vi "ziModGetIntegerData.vi"(8 "Error In":errorcluster, 10 "ModResults":T3, 11 "ModHandle In":T7 {"ModHandle" format="0x%08x"; "Conn" format="0x%08x"}) -> (0 "Error Out":errorcluster, 1 "ModIntegerDataGrid":T1[](array[typedef]), 2 "ModIntegerData":T2[](array[typedef]), 3 "ModHandle Out":T7 {"ModHandle" format="0x%08x"; "Conn" format="0x%08x"}, 4 "Value":i64[](array[numeric]))   [LabVIEW 2009, in "Zurich Instruments LabOne.lvlib"]
doc: "Use this vi to get IntegerData from a ModResult returned from ziModGetNextNode.vi. It return an array of IntegerData."
uses:
  <instrlib>/Zurich Instruments LabOne/Zurich Instruments LabOne.lvlib
  <instrlib>/Zurich Instruments LabOne/Public/Modules/ziTypeModHandle.ctl
  <instrlib>/Zurich Instruments LabOne/Public/Modules/ziTypeModResults.ctl
  <instrlib>/Zurich Instruments LabOne/Public/Data/ziTypePollType.ctl
  <instrlib>/Zurich Instruments LabOne/Public/Modules/ziTypeModSWTriggerHeader.ctl
  <instrlib>/Zurich Instruments LabOne/Public/Modules/ziTypeModSweeperHeader.ctl
  <instrlib>/Zurich Instruments LabOne/Public/Data/ziTypeIntegerDataTS.ctl
  <instrlib>/Zurich Instruments LabOne/Public/Data/ziTypeIntegerDataTSGrid.ctl
  <instrlib>/Zurich Instruments LabOne/Private/ziLV32.dll
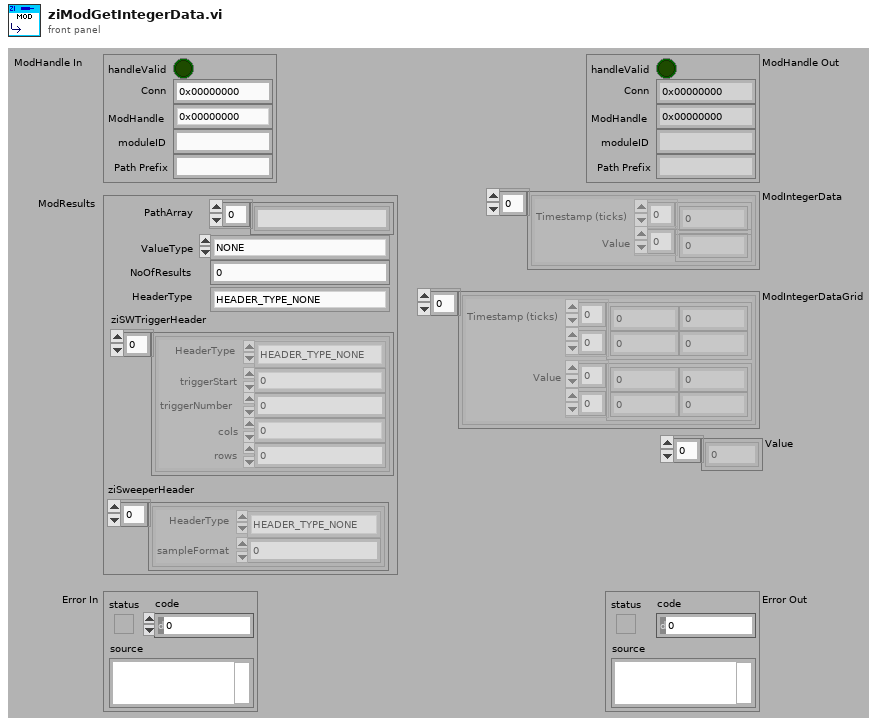
[diagram p1: front panel]
types:
  T1 = typedef "ziTypeIntegerDataTSGrid.ctl" = cluster{"Timestamp (ticks)":u64[][], "Value":i64[][]}
  T2 = typedef "Zurich Instruments LabOne.lvlib/ziTypeIntegerDataTS.ctl" = cluster{"Timestamp (ticks)":u64[], "Value":i64[]}
  T3 = typedef "Zurich Instruments LabOne.lvlib/ziTypeModResults.ctl" = cluster{"PathArray":string[], "ValueType":T4, "NoOfResults":u64, "HeaderType":enum16{"HEADER_TYPE_NONE", "HEADER_TYPE_SWTRIGGER", "HEADER_TYPE_SWEEPER"}, "ziSWTriggerHeader":T5[], "ziSweeperHeader":T6[]}
  T4 = typedef "Zurich Instruments LabOne.lvlib/ziTypePollType.ctl" = enum16{"NONE", "DOUBLE_DATA", "INTEGER_DATA", "DEMOD_SAMPLE", "SCOPE_WAVE_HF2", "AUXIN_SAMPLE", "DIO_SAMPLE", "BYTE_ARRAY", "PWA_WAVE", "9", "10", "11", "12", "13", "14", "15", "TREE_CHANGE_DEPRI", "17", "ERROR", "19", "20", "21", "22", "23", "24", "25", "26", "27", "28", "29", "30", "31", "DOUBLE_DATA_TS", "INTEGER_DATA_TS", "34", "SCOPE_WAVE", "36", "37", "BYTE_ARRAY_TS", "39", "40", "41", "42", "43", "44", "45", "CNT_DATA", "47", "TREE_CHANGE", "49", "50", "51", "52", "53", "54", "55", "56", "57", "58", "59", "60", "61", "62", "63", "SWEEPER_DATA", "SPECTRUM_DATA", "ADVISOR_DATA", "67", "IMP_DATA"}
  T5 = typedef "Zurich Instruments LabOne.lvlib/ziTypeModSWTriggerHeader.ctl" = cluster{"HeaderType":enum8{"HEADER_TYPE_NONE", "HEADER_TYPE_SWTRIGGER", "HEADER_TYPE_SWEEPER"}, "triggerStart":u64, "triggerNumber":u64, "cols":u32, "rows":u32}
  T6 = typedef "Zurich Instruments LabOne.lvlib/ziTypeModSweeperHeader.ctl" = cluster{"HeaderType":enum8{"HEADER_TYPE_NONE", "HEADER_TYPE_SWTRIGGER", "HEADER_TYPE_SWEEPER"}, "sampleFormat":u8}
  T7 = typedef "Zurich Instruments LabOne.lvlib/ziTypeModHandle.ctl" = cluster{"handleValid":bool, "Conn":u64, "ModHandle":u64, "moduleID":string, "Path Prefix":string}
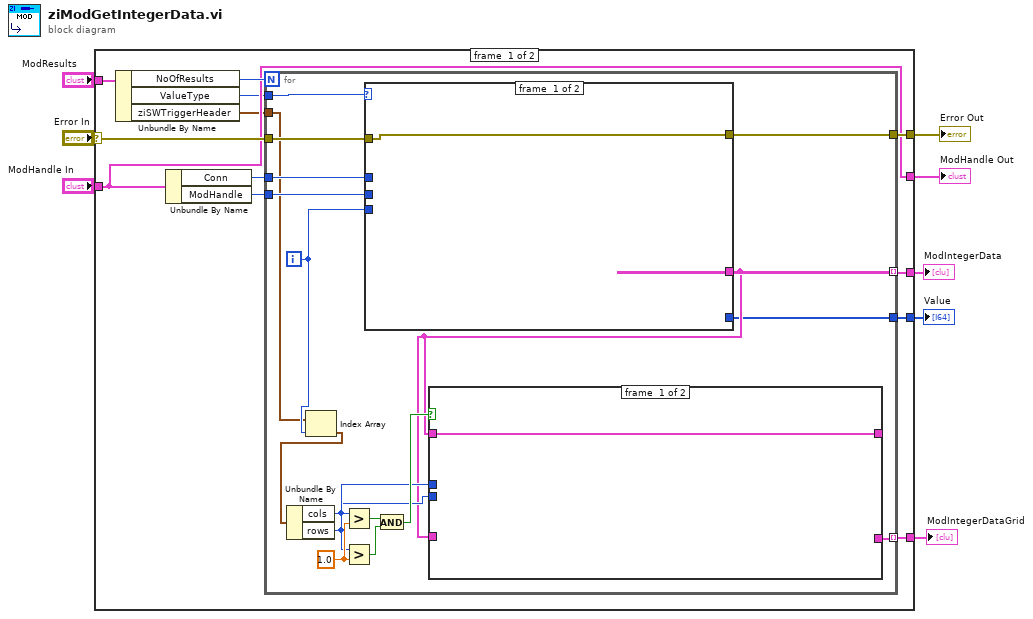
[diagram p0: block diagram]
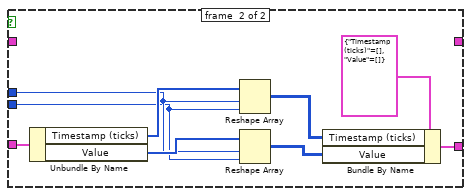
[diagram p2: hidden frame]
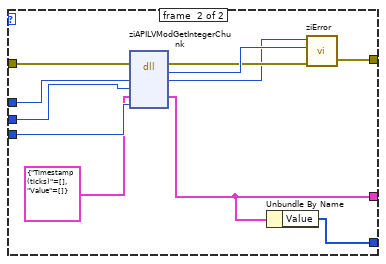
[diagram p3: hidden frame]
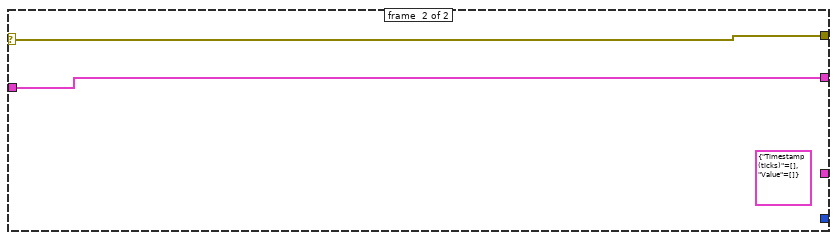
[diagram p4: hidden frame]
diagram:
  n1 = case shown="No Error" "Error In" {
    selector: "Error In" -> [w15 w60]
    tunnel: [w16 w60] -> w4
    tunnel: [w14 w61] -> w7
    tunnel: "ModHandle In" -> [w14 w61]
    tunnel: "ModResults" -> [w18 _]
    tunnel: [w13 _] -> w3
    tunnel: [w10 _] -> w2
    tunnel: [w9 _] -> w1
    frame #0 {
      n2 = Unbundle By Name(w18) -> ("NoOfResults"=w17:u64, "ValueType"=w12:T4, "ziSWTriggerHeader"=w11:T5[])
      n3 = Unbundle By Name(w14) -> ("Conn"=w20:u64, "ModHandle"=w19:u64)
      n4 = for {
        N: w17 -> [_]
        tunnel: w20 -> [w37]
        tunnel: w19 -> [w36]
        tunnel: [w35] -> w16
        tunnel: w15 -> [w34]
        tunnel: [w26] -> w13 mode=indexing
        tunnel: w12 -> [w33]
        tunnel: w11 -> [w22]
        tunnel: [w25] -> w10 mode=indexing
        tunnel: [w21] -> w9
        i -> [w23]
        w32 = 1.0 ("y")
        n5 = Index Array(array=w22, index=w23) -> (element=w24:T5)
        n6 = Unbundle By Name(w24) -> ("cols"=w27:u32, "rows"=w28:u32)
        n7 = Greater?(x=w27, y=w32) -> (0:w30:bool)
        n8 = Greater?(x=w28, y=w32) -> (0:w31:bool)
        n9 = case shown="\"INTEGER_DATA\"" w33 {
          tunnel: w37 -> [_ w59]
          tunnel: w36 -> [_ w58]
          tunnel: w23 -> [_ w57]
          tunnel: [w48 w56] -> w35
          tunnel: w34 -> [w48 w53]
          tunnel: [_ w50] -> w26
          tunnel: [_ w49] -> w21
          frame #0 {
          }
          frame #1 {
            n10 = dll-call lib="C:/Program Files (x86)/National Instruments/LabVIEW 2009/instr.lib/Zurich Instruments LabOne/Private/ziLV*.*" fn="ziAPILVModGetIntegerChunk"(error in=w53, "Conn"=w59, "ModHandle"=w58, "IntegerData"=T2 {"Timestamp (ticks)"=[], "Value"=[]} ("IntegerSample 3"), "chunk_idx"=w57) -> (error out=w54:errorcluster, "return type"=w55:u32, "Conn"=w52:u64, "IntegerData"=w50:T2)  [unwired: 4 in, 1 out]
            n11 = Unbundle By Name(w50) -> ("Value"=w49:i64[])
            n12 = call <instrlib>:"ziError.vi"("Conn"=w52, "ziErrorCode"=w55, "Error In"=w54) -> ("Error Out"=w56:errorcluster)  [unwired: 2 in, 1 out]
          }
        }
        n13 = And(x=w30, y=w31) -> (x .and. y?=w29:bool)
        n14 = case shown="True" w29 {
          tunnel: w26 -> [_ w47]
          tunnel: w26 -> [w38 _]
          tunnel: [w38 _] -> _
          tunnel: w28 -> [_ w44]
          tunnel: w27 -> [_ w42]
          tunnel: [_ w43] -> w25
          frame #0 {
          }
          frame #1 {
            n15 = Unbundle By Name(w47) -> ("Timestamp (ticks)"=w46:u64[], "Value"=w45:i64[])
            n16 = Reshape Array(w46, w44, w42) -> (w41:u64[][])
            n17 = Reshape Array(w45, w44, w42) -> (w40:i64[][])
            n18 = Bundle By Name(cluster=T1 {"Timestamp (ticks)"=[], "Value"=[]} ("IntegerData"), "Timestamp (ticks)"=w41, "Value"=w40) -> (w43:T1)
          }
        }
      }
    }
    frame #1 {
      (unwired) T2 {"Timestamp (ticks)"=[], "Value"=[]} ("IntegerSample 2")
    }
  }
  "Error Out" <- w4
  "ModHandle Out" <- w7
  "ModIntegerData" <- w3
  "ModIntegerDataGrid" <- w2
  "Value" <- w1
